vi "svx_DAQ_LoadFromXML.vi"(7 "XControl Ref":refnum<vi>, 8 "error in (no error)":errorcluster, 9 "cluster":T2, 10 "Display State In":T3={"Channel Info Array"=[], "Timing Mode"=enum."Time", "Timing Control 1"=25600.0, "Timing Control 2"=2560.0, "Timing Control 3"=16, "Timing Indicator 1"=0.1, "Reference Visible?"=FALSE, "Reference Type"=enum."<none>", "Tachometer Channel"="", "Tach Pulses Per Rev"=1, "Tach Direction"=enum."CW", "Tach Slope"=enum."Rising", "Tach Threshold"=0.0, "Trigger Channel"="", "Trigger Level"=20.0, "Pretrigger Samples"=1, "Trigger Slope"=enum."Falling", "Trigger Hysteresis"=0.0, "Logging Visible?"=FALSE, "Enable Logging"=FALSE, "Logfile Path"=path "c:/test.tdms"} caption="State" {"Timing Control 2" format="%#_6f"; "Channel Info Array"."Max" min=0.0 format="± %^#_4g"; "Channel Info Array"."Channel Type" items=["Voltage (V)"=0, "Charge (C)"=9, "-"=99, "SPL (Pa)"=3, "Force (lbf)"=6, "Force (N)"=1, "Acceleration (g) - IEPE"=2, "Acceleration (g) - Charge"=12, "Acceleration (g) - 4 wire DC Voltage"=22, "Velocity (in/s)"=7, "Velocity (mm/s)"=8, "Prox Probe (mil)"=4, "Prox Probe (mm)"=5]}, 11 "Data In":T1) -> (0 "error out":errorcluster, 2 "Display State Out":T3={"Channel Info Array"=[], "Timing Mode"=enum."Time", "Timing Control 1"=25600.0, "Timing Control 2"=2560.0, "Timing Control 3"=16, "Timing Indicator 1"=0.1, "Reference Visible?"=FALSE, "Reference Type"=enum."<none>", "Tachometer Channel"="", "Tach Pulses Per Rev"=1, "Tach Direction"=enum."CW", "Tach Slope"=enum."Rising", "Tach Threshold"=0.0, "Trigger Channel"="", "Trigger Level"=20.0, "Pretrigger Samples"=1, "Trigger Slope"=enum."Falling", "Trigger Hysteresis"=0.0, "Logging Visible?"=FALSE, "Enable Logging"=FALSE, "Logfile Path"=path "c:/test.tdms"} caption="State" {"Timing Control 2" format="%#_6f"; "Channel Info Array"."Max" min=0.0 format="± %^#_4g"; "Channel Info Array"."Channel Type" items=["Voltage (V)"=0, "Charge (C)"=9, "-"=99, "SPL (Pa)"=3, "Force (lbf)"=6, "Force (N)"=1, "Acceleration (g) - IEPE"=2, "Acceleration (g) - Charge"=12, "Acceleration (g) - 4 wire DC Voltage"=22, "Velocity (in/s)"=7, "Velocity (mm/s)"=8, "Prox Probe (mil)"=4, "Prox Probe (mm)"=5]}, 3 "Data Out":T1, 4 "State and Data Changed?":bool=TRUE)   [LabVIEW 2017, in "SVX NI-DAQmx AI Configuration XControl.xctl"]
uses:
  <vilib>/addons/Sound and Vibration/svt_DAQmx/Configuration XControl/SVX NI-DAQmx AI Configuration XControl.xctl
  <vilib>/addons/Sound and Vibration/svt_DAQmx/Configuration XControl/SubVIs/svx_DAQ_State.ctl
  <vilib>/addons/Sound and Vibration/svt_DAQmx/Configuration XControl/Controls/svx_DAQ_ChannelInfo.ctl
  <vilib>/addons/Sound and Vibration/svt_DAQmx/Configuration XControl/Controls/svx_DAQ_ChannelType.ctl
  <vilib>/addons/Sound and Vibration/svt_DAQmx/Configuration XControl/Controls/svx_DAQ_Coupling.ctl
  <vilib>/addons/Sound and Vibration/svt_DAQmx/Configuration XControl/Controls/svx_DAQ_Excitation.ctl
  <vilib>/addons/Sound and Vibration/svt_DAQmx/Configuration XControl/Controls/svx_DAQ_TimingType.ctl
  <vilib>/addons/Sound and Vibration/svt_DAQmx/Configuration XControl/Controls/svx_DAQ_ReferenceType.ctl
  <vilib>/addons/Sound and Vibration/svt_DAQmx/Configuration XControl/Controls/svx_DAQ_RotationDirection.ctl
  <vilib>/addons/Sound and Vibration/svt_DAQmx/Configuration XControl/Controls/svx_DAQ_Tach_Slope.ctl
  <vilib>/addons/Sound and Vibration/svt_DAQmx/Configuration XControl/Controls/svx_DAQ_Trigger_Slope.ctl
  <vilib>/addons/Sound and Vibration/svt_DAQmx/Configuration XControl/SubVIs/svx_DAQ_Data.ctl
  <vilib>/addons/Sound and Vibration/svt_DAQmx/Configuration XControl/Controls/svx_DAQ_ControlRefs.ctl
  <vilib>/Utility/xml.llb/Read From XML File(string).vi
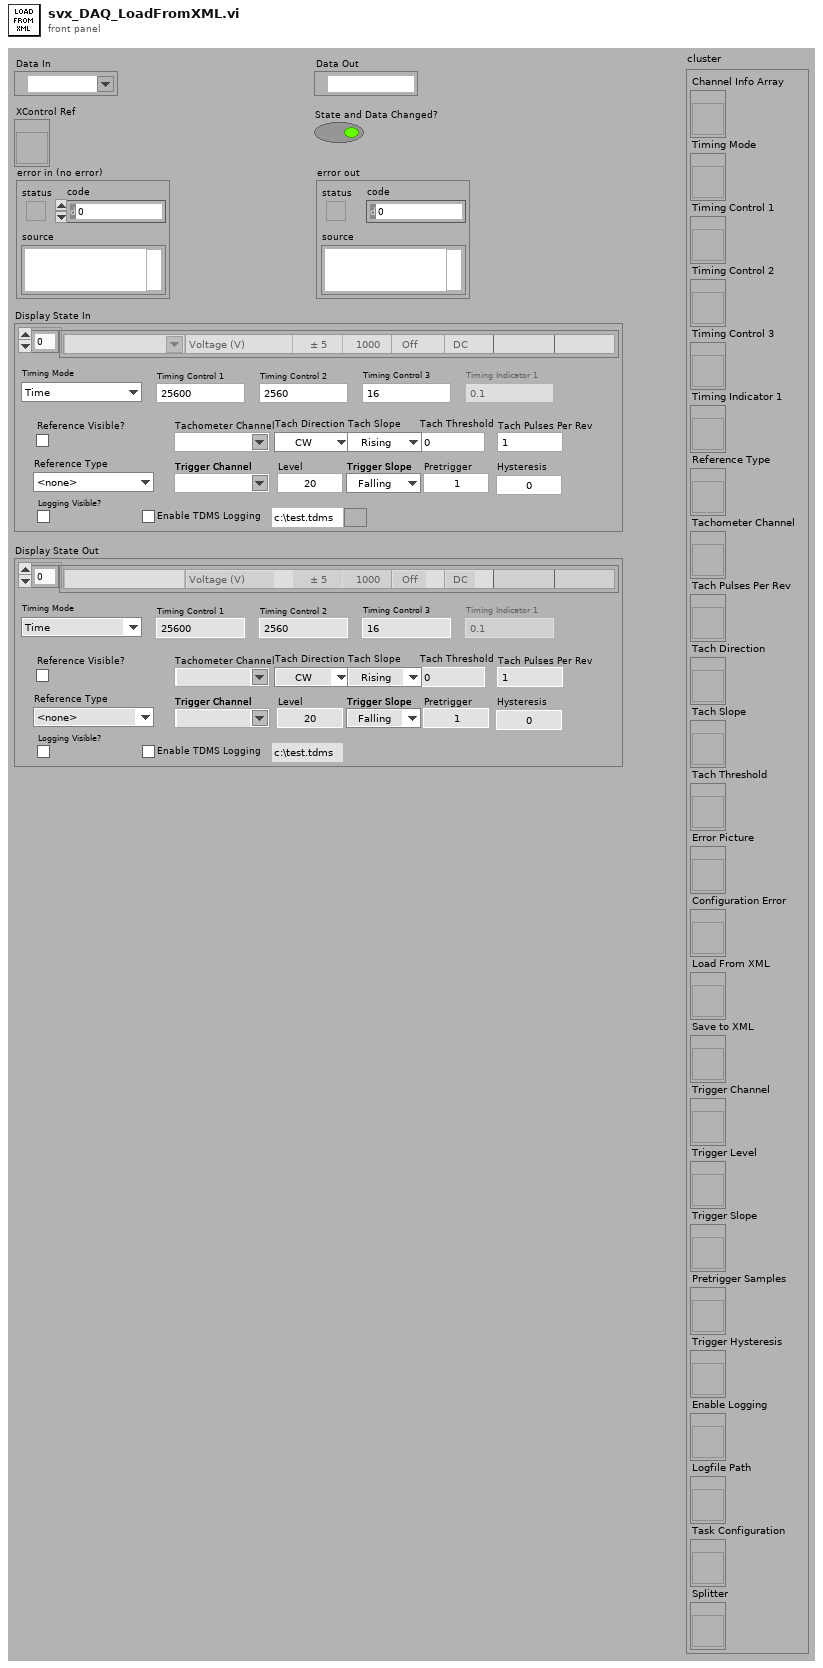
[diagram p1: front panel]
types:
  T1 = typedef "SVX NI-DAQmx AI Configuration XControl.xctl/svx_DAQ_Data.ctl" = refnum<k21>
  T2 = typedef "SVX NI-DAQmx AI Configuration XControl.xctl/svx_DAQ_ControlRefs.ctl" = cluster{"Channel Info Array":refnum<vi>, "Timing Mode":refnum<vi>, "Timing Control 1":refnum<vi>, "Timing Control 2":refnum<vi>, "Timing Control 3":refnum<vi>, "Timing Indicator 1":refnum<vi>, "Reference Type":refnum<vi>, "Tachometer Channel":refnum<vi>, "Tach Pulses Per Rev":refnum<vi>, "Tach Direction":refnum<vi>, "Tach Slope":refnum<vi>, "Tach Threshold":refnum<vi>, "Error Picture":refnum<vi>, "Configuration Error":refnum<vi>, "Load From XML":refnum<vi>, "Save to XML":refnum<vi>, "Trigger Channel":refnum<vi>, "Trigger Level":refnum<vi>, "Trigger Slope":refnum<vi>, "Pretrigger Samples":refnum<vi>, "Trigger Hysteresis":refnum<vi>, "Enable Logging":refnum<vi>, "Logfile Path":refnum<vi>, "Task Configuration":refnum<vi>, "Splitter":refnum<vi>}
  T3 = typedef "SVX NI-DAQmx AI Configuration XControl.xctl/svx_DAQ_State.ctl" = cluster{"Channel Info Array":T4[], "Timing Mode":T8, "Timing Control 1":dbl, "Timing Control 2":dbl, "Timing Control 3":i32, "Timing Indicator 1":dbl, "Reference Visible?":bool, "Reference Type":T9, "Tachometer Channel":string, "Tach Pulses Per Rev":i32, "Tach Direction":T10, "Tach Slope":T11, "Tach Threshold":dbl, "Trigger Channel":string, "Trigger Level":dbl, "Pretrigger Samples":i32, "Trigger Slope":T12, "Trigger Hysteresis":dbl, "Logging Visible?":bool, "Enable Logging":bool, "Logfile Path":path}
  T4 = typedef "SVX NI-DAQmx AI Configuration XControl.xctl/svx_DAQ_ChannelInfo.ctl" = cluster{"Initialized?":bool, "DAQmx Channel":tag, "Channel Type":T5, "Max":dbl, "Sensitivity":dbl, "Excitation":bool, "Coupling":T6, "Location":string, "Orientation":string, "excitation":T7}
  T5 = typedef "SVX NI-DAQmx AI Configuration XControl.xctl/svx_DAQ_ChannelType.ctl" = u16
  T6 = typedef "SVX NI-DAQmx AI Configuration XControl.xctl/svx_DAQ_Coupling.ctl" = enum16{"AC", "DC"}
  T7 = typedef "svx_DAQ_Excitation.ctl" = enum16{"Off", "Min", "Max"}
  T8 = typedef "SVX NI-DAQmx AI Configuration XControl.xctl/svx_DAQ_TimingType.ctl" = enum16{"Time", "Frequency", "Order"}
  T9 = typedef "SVX NI-DAQmx AI Configuration XControl.xctl/svx_DAQ_ReferenceType.ctl" = enum16{"<none>", "Analog Tachometer", "Analog SW Trigger"}
  T10 = typedef "SVX NI-DAQmx AI Configuration XControl.xctl/svx_DAQ_RotationDirection.ctl" = enum16{"CW", "CCW"}
  T11 = typedef "SVX NI-DAQmx AI Configuration XControl.xctl/svx_DAQ_Tach_Slope.ctl" = enum16{"Rising", "Falling"}
  T12 = typedef "SVX NI-DAQmx AI Configuration XControl.xctl/svx_DAQ_Trigger_Slope.ctl" = enum16{"Falling", "Rising"}
  T13 = cluster{"Channel Info Array":cluster{"Initialized?":bool, "DAQmx Channel":tag, "Channel Type":T5, "Max":dbl, "Sensitivity":dbl, "IEPE":bool, "Coupling":T6, "Location":string, "Orientation":string}[], "Timing Mode":T8, "Timing Control 1":dbl, "Timing Control 2":dbl, "Timing Control 3":i32, "Timing Indicator 1":dbl, "Reference Visible?":bool, "Reference Type":T9, "Tachometer Channel":string, "Tach Pulses Per Rev":i32, "Tach Direction":T10, "Tach Slope":T11, "Tach Threshold":dbl, "Trigger Channel":string, "Trigger Level":dbl, "Pretrigger Samples":i32, "Trigger Slope":T12, "Trigger Hysteresis":dbl, "Logging Visible?":bool, "Enable Logging":bool, "Logfile Path":path}
  T14 = cluster{"Channel Info Array":cluster{"Initialized?":bool, "DAQmx Channel":tag, "Channel Type":enum16{"Voltage (V)", "Force (N)", "Acceleration (g)", "SPL (Pa)", "Prox Probe (mil)", "Prox Probe (mm)"}, "Max":dbl, "Sensitivity":dbl, "IEPE":bool, "Coupling":enum16{"AC", "DC"}, "Location":string, "Orientation":string}[], " Mode ":enum16{"Time", "Frequency", "Order"}, "Timing Control 1":dbl, "Timing Control 2":dbl, "Timing Control 3":i32, "Timing Indicator 1":dbl, "Tachometer?":bool, "Pulses Per Rev":i32, "Direction":enum16{"CW", "CCW"}, "Slope":enum16{"Rising", "Falling"}, "Threshold":dbl, "Tachometer Channel":string}
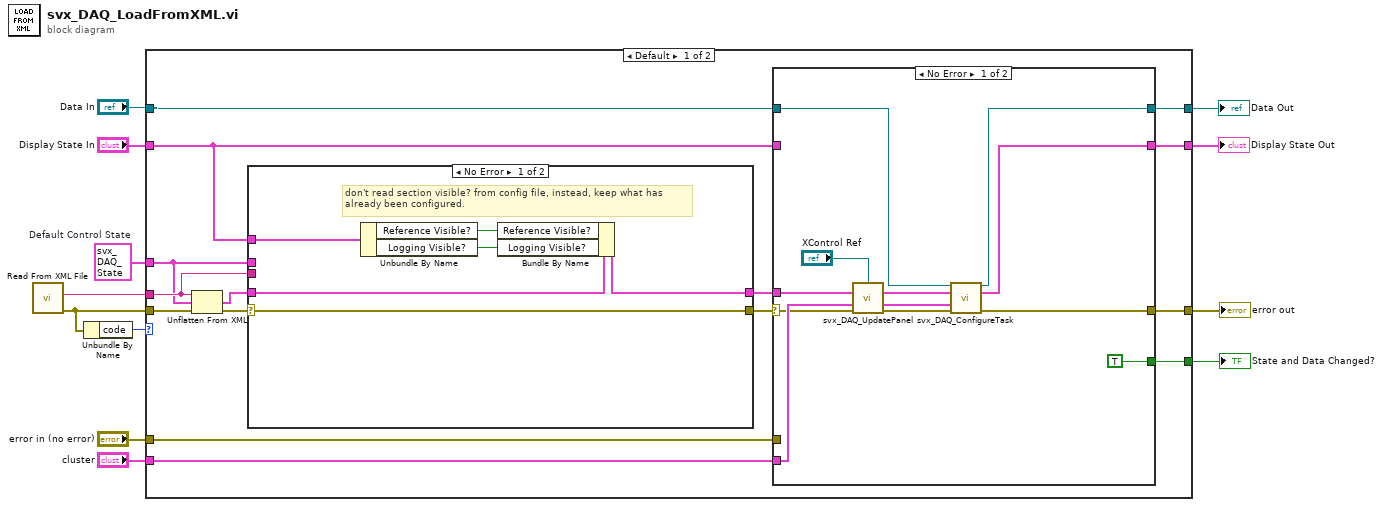
[diagram p0: block diagram]
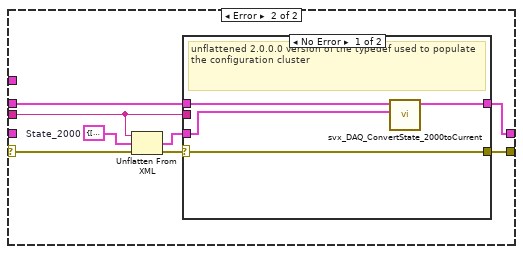
[diagram p2: hidden frame]
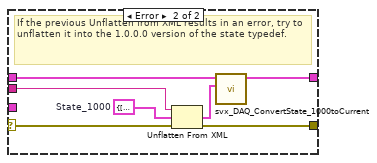
[diagram p3: hidden frame]
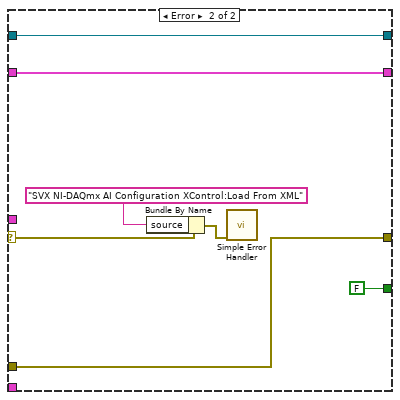
[diagram p4: hidden frame]
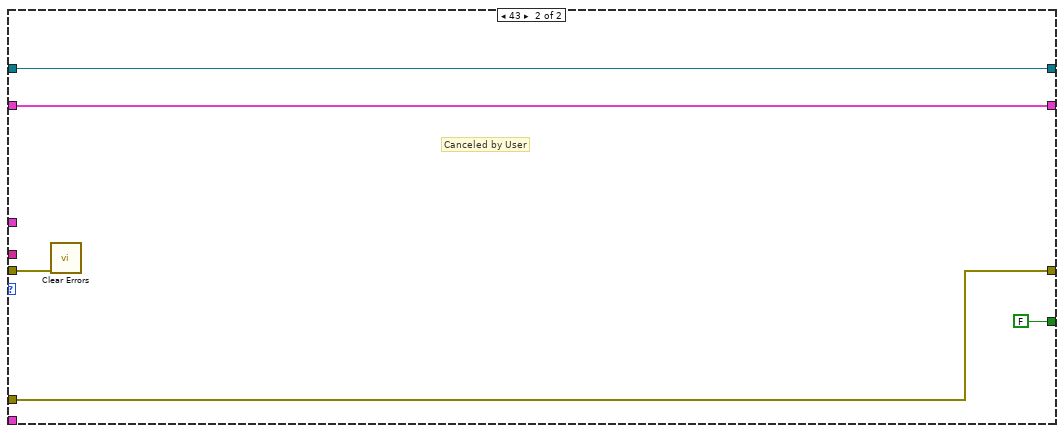
[diagram p5: hidden frame]
diagram:
  w1 = T3 {"Channel Info Array"=[], "Timing Mode"=enum."Time", "Timing Control 1"=25600.0, "Timing Control 2"=2560.0, "Timing Control 3"=16, "Timing Indicator 1"=0.1, "Reference Visible?"=TRUE, "Reference Type"=enum."<none>", "Tachometer Channel"="", "Tach Pulses Per Rev"=1, "Tach Direction"=enum."CW", "Tach Slope"=enum."Rising", "Tach Threshold"=0.0, "Trigger Channel"="", "Trigger Level"=1.0, "Pretrigger Samples"=20, "Trigger Slope"=enum."Rising", "Trigger Hysteresis"=0.0, "Logging Visible?"=TRUE, "Enable Logging"=FALSE, "Logfile Path"=path ""}  # Default Control State
  n1 = call-poly <vilib>:"Read From XML File.vi"() -> ("error out"=w11:errorcluster, "XML Elements"=w12:string)  [unwired: 9 in, 1 out]
  n2 = Unbundle By Name(w11) -> ("code"=w10:i32)
  n3 = case shown="Default" w10 {
    tunnel: [w22 w75] -> w3
    tunnel: w1 -> [w15 _]
    tunnel: w12 -> [w16 _]
    tunnel: w11 -> [w27 w76]
    tunnel: "error in (no error)" -> [w21 w75]
    tunnel: "cluster" -> [w26 _]
    tunnel: "Display State In" -> [w13 w74]
    tunnel: "Data In" -> [w25 w73]
    tunnel: [w24 w73] -> w5
    tunnel: [w23 w74] -> w4
    tunnel: [w20 FALSE] -> w2
    frame Default {
      n4 = Unflatten From XML(xml string=w16, type=w15, error in (no error)=w27) -> (value=w14:T3, error out=w19:errorcluster)
      n5 = case shown="No Error" w19 {
        selector: w19 -> [w33 w39]
        tunnel: [w31 w40] -> w18
        tunnel: [w33 w41] -> w17
        tunnel: w16 -> [_ w37]
        tunnel: w15 -> [_ w36]
        tunnel: w14 -> [w32 _]
        tunnel: w13 -> [w30 _]
        frame No Error {
          # "don't read section visible? from config file, instead, keep what has\nalready been configured."
          n6 = Unbundle By Name(w30) -> ("Reference Visible?"=w29:bool, "Logging Visible?"=w28:bool)
          n7 = Bundle By Name(cluster=w32, "Reference Visible?"=w29, "Logging Visible?"=w28) -> (w31:T3)
        }
        frame Error {
          w34 = T13 {"Channel Info Array"=[], "Timing Mode"=enum."Time", "Timing Control 1"=0.0, "Timing Control 2"=0.0, "Timing Control 3"=0, "Timing Indicator 1"=0.0, "Reference Visible?"=FALSE, "Reference Type"=enum."<none>", "Tachometer Channel"="", "Tach Pulses Per Rev"=0, "Tach Direction"=enum."CW", "Tach Slope"=enum."Rising", "Tach Threshold"=0.0, "Trigger Channel"="", "Trigger Level"=0.0, "Pretrigger Samples"=0, "Trigger Slope"=enum."Falling", "Trigger Hysteresis"=0.0, "Logging Visible?"=FALSE, "Enable Logging"=FALSE, "Logfile Path"=path ""}  # State_2000
          n8 = Unflatten From XML(xml string=w37, type=w34, error in (no error)=w39) -> (value=w35:T13, error out=w38:errorcluster)
          n9 = case shown="No Error" w38 {
            selector: w38 -> [w43 w47]
            tunnel: w37 -> [_ w52]
            tunnel: [w43 w51] -> w41
            tunnel: w36 -> [w45 w50]
            tunnel: [w44 w49] -> w40
            tunnel: w35 -> [w42 _]
            frame No Error {
              # "unflattened 2.0.0.0 version of the typedef used to populate the configuration cluster"
              n10 = call <vilib>:"svx_DAQ_ConvertState_2000toCurrent.vi"("State_2000"=w42, "Default Control State in"=w45) -> ("Default Control State out"=w44:T3)  [unwired: 9 in]
            }
            frame Error {
              w46 = T14 {"Channel Info Array"=[], " Mode "=enum."Time", "Timing Control 1"=25600.0, "Timing Control 2"=2560.0, "Timing Control 3"=16, "Timing Indicator 1"=0.1, "Tachometer?"=FALSE, "Pulses Per Rev"=0, "Direction"=enum."CCW", "Slope"=enum."Rising", "Threshold"=0.0, "Tachometer Channel"=""}  # State_1000
              # "If the previous Unflatten from XML results in an error, try to unflatten it into the 1.0.0.0 version of the state typedef."
              n11 = Unflatten From XML(xml string=w52, type=w46, error in (no error)=w47) -> (value=w48:T14, error out=w51:errorcluster)
              n12 = call <vilib>:"svx_DAQ_ConvertState_1000toCurrent.vi"("saved state (version 1.0.0.0)"=w48, "current state template"=w50) -> ("Default Control State out"=w49:T3)  [unwired: 9 in]
            }
          }
        }
      }
      n13 = case shown="No Error" w17 {
        selector: w17 -> [w55 w67]
        tunnel: w18 -> [w64 _]
        tunnel: [w63 w71] -> w24
        tunnel: [w62 w66] -> w22
        tunnel: w26 -> [w59 _]
        tunnel: [w57 w70] -> w23
        tunnel: w25 -> [w56 w71]
        tunnel: w13 -> [_ w70]
        tunnel: w21 -> [_ w66]
        tunnel: [TRUE FALSE] -> w20
        frame No Error {
          n14 = call <vilib>:"svx_DAQ_UpdatePanel.vi"("XControl Ref"="XControl Ref", "State"=w64, "cluster"=w59, "error in (no error)"=w55) -> ("State Out"=w60:T3, "cluster"=w58:T2, "error out"=w61:errorcluster)  [unwired: 9 in]
          n15 = call <vilib>:"svx_DAQ_ConfigureTask.vi"("Task In"=w56, "Display State In"=w60, "cluster"=w58, "error in"=w61) -> ("task out"=w63:refnum<k21>, "Display State Out"=w57:T3, "error out"=w62:errorcluster)  [unwired: 8 in, 1 out]
        }
        frame Error {
          n16 = Bundle By Name(cluster=w67, "source"="SVX NI-DAQmx AI Configuration XControl:Load From XML") -> (w69:errorcluster)
          n17 = call <vilib>:"Simple Error Handler.vi"("error in (no error)"=w69) -> ()  [unwired: 4 in, 5 out]
        }
      }
    }
    frame 43 {
      # "Canceled by User"
      n18 = call <vilib>:"Clear Errors.vi"("error in (no error)"=w76) -> ()  [unwired: 5 in, 2 out]
    }
  }
  "error out" <- w3
  "Display State Out" <- w4
  "Data Out" <- w5
  "State and Data Changed?" <- w2
